vi "Get Attributes.vi"(8 "error in (no error)":errorcluster, 11 "Pulse Train in":refnum<class "Pulse Train.lvclass">) -> (0 "error out":errorcluster, 2 "Attributes":T1, 3 "Pulse Train out":refnum<class "Pulse Train.lvclass">)   [LabVIEW 2020, in "Pulse Train.lvclass"]
uses:
  Pulse Train.lvclass
  Waveform/Attributes.ctl
  Waveform/Waveform.lvclass
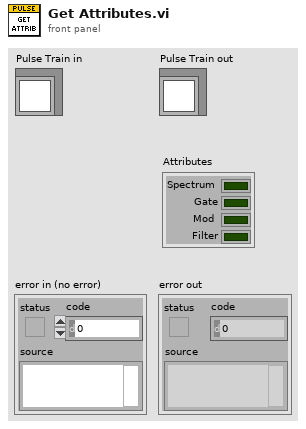
[diagram p1: front panel]
types:
  T1 = typedef "Waveform.lvclass/Attributes.ctl" = cluster{"Spectrum":bool, "Gate":bool, "Mod":bool, "Filter":bool}
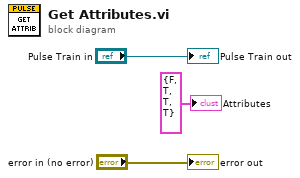
[diagram p0: block diagram]
diagram:
  "error out" <- "error in (no error)"
  "Pulse Train out" <- "Pulse Train in"
  "Attributes" <- T1 {"Spectrum"=FALSE, "Gate"=TRUE, "Mod"=TRUE, "Filter"=TRUE} ("Attributes")
